vi "Periodic Tasks.vi"(8 "error in":errorcluster) -> ()   [LabVIEW 2014]
doc: "This VI runs in parallel to other tasks. It can contain as many user-defined periodic loops as you need. These can carry out PID or other sorts of timed response."
uses:
  <vilib>/Rock Robotics/SystemInterfaces/Utilities/FPGA_UtilitiesLED Source.ctl
  <vilib>/Rock Robotics/SystemInterfaces/Utilities/FPGA_UtilitiesLED State.ctl
  <vilib>/Rock Robotics/WPI/Compressor/WPI_CompressorGetSetRefNum.vi
  Robot Global Data.vi
  <vilib>/Rock Robotics/WPI/Relay/WPI_RelayValue.ctl
panel:
  out "Accel":dbl[](graph)=[0.0, 0.004] caption="Acceleration"
  in  "Blink Time (ms)":i32=2000
  in  "Thresh":dbl=1.0 caption="Acceleration Threshold"
  in  "Blink Speed":dbl=157.0 format="%#_13g"
  out "Color":u32(colorbox)=16728064
  in  "Speed":dbl=5.0 format="%#_13g"
  in  "Saturation":dbl(slide)=1.0 scale=0.0..1.0
  in  "Value":dbl(slide)=1.0 scale=0.0..1.0
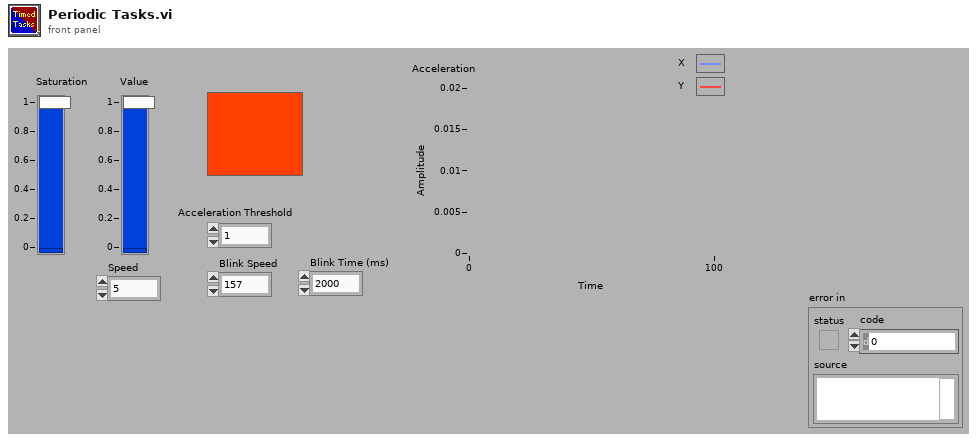
[diagram p1: front panel]
types:
  T1 = typedef "LEDStripRef.ctl" = cluster{"PWM Rate (Hz)":sgl, "Max Duty Cycle":sgl, "DigitalOutputRed":T2, "DigitalOutputGreen":T2, "DigitalOutputBlue":T2, "DevStatus":errorcluster}
  T2 = typedef "WPI_DigitalOutputDevRef.ctl" = cluster{"Digital Module":T3, "DIO Channel":T4, "DevStatus":errorcluster}
  T3 = typedef "FPGA_TypedefDigitalModule.ctl" = enum16{"Digital Module 1", "Digital Module 2"}
  T4 = typedef "FPGA_DIOChannel.ctl" = enum8{"DIO 1", "DIO 2", "DIO 3", "DIO 4", "DIO 5", "DIO 6", "DIO 7", "DIO 8", "DIO 9", "DIO 10", "DIO 11", "DIO 12", "DIO 13", "DIO 14", "Invalid"}
  T5 = typedef "WPI_I2CDevRef.ctl" = cluster{"DevStatus":errorcluster, "Digital Module":T3, "Device Address":u8}
  T6 = typedef "WPI_DigitalInputDevRef.ctl" = cluster{"DevStatus":errorcluster, "DIO Channel":T4, "Digital Module":T3}
  T7 = typedef "WPI_DriverStationRobotMode2.ctl" = enum16{"Autonomous Disabled", "Autonomous Enabled", "Teleop Disabled", "Teleop Enabled", "Disconnected", "Finish", "Test Disabled", "Test Enabled"}
  T8 = typedef "WPI_DriverStationAllianceInfo.ctl" = enum16{"Red", "Blue", "Invalid"}
  T9 = typedef "FPGA_UtilitiesLED State.ctl" = enum16{"Off", "On", "Toggle"}
  T10 = typedef "FPGA_UtilitiesLED Source.ctl" = enum16{"User LED", "FPGA LED"}
  T11 = typedef "WPI_CompressorDevRef.ctl" = cluster{"DevStatus":errorcluster, "DigitalInputDevRef":T6, "RelayDevRef":T12}
  T12 = typedef "WPI_RelayDevRef.ctl" = cluster{"DevStatus":errorcluster, "Relay Channel":T13, "Digital Module":T3, "Relay Direction":T14}
  T13 = typedef "FPGA_DIORelayChannel.ctl" = enum8{"Relay 1", "Relay 2", "Relay 3", "Relay 4", "Relay 5", "Relay 6", "Relay 7", "Relay 8", "Invalid"}
  T14 = typedef "WPI_RelayDirection.ctl" = enum16{"Both directions", "Forward only", "Reverse only"}
  T15 = typedef "WPI_RelayValue.ctl" = enum16{"Off", "On", "Forward", "Reverse"}
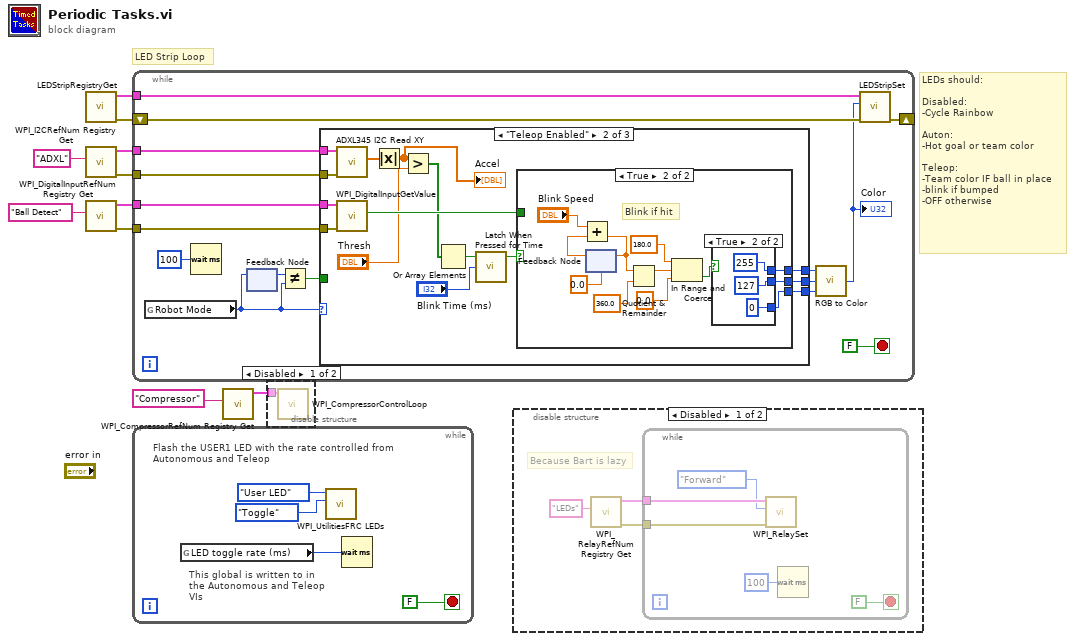
[diagram p0: block diagram]
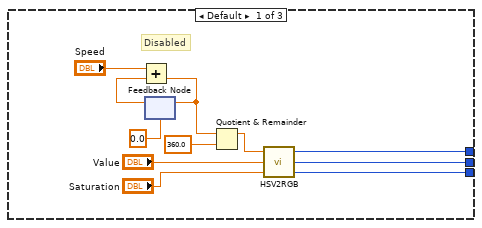
[diagram p4: hidden frame]
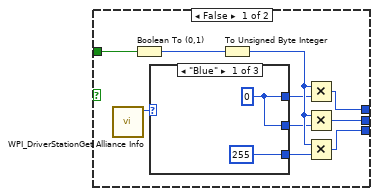
[diagram p5: hidden frame]
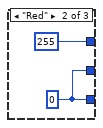
[diagram p6: hidden frame]
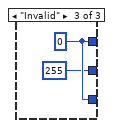
[diagram p7: hidden frame]
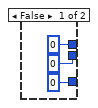
[diagram p8: hidden frame]
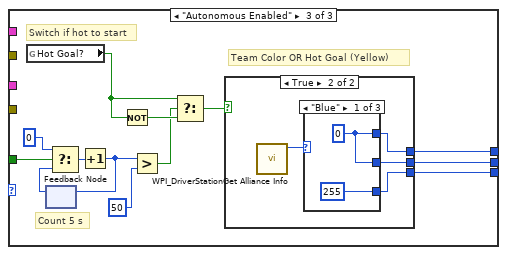
[diagram p9: hidden frame]
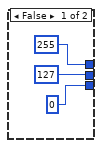
[diagram p10: hidden frame]
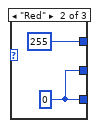
[diagram p11: hidden frame]
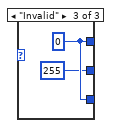
[diagram p12: hidden frame]
diagram:
  # "LEDs should:\n\nDisabled:\n-Cycle Rainbow\n\nAuton: \n-Hot goal or team color\n\nTeleop:\n-Team color IF ball in place\n-blink if bumped\n-OFF otherwise"
  # "LED Strip Loop"
  n1 = call "LEDStripRegistryGet.vi"() -> ("error out"=w7:errorcluster, "LEDStripRef out"=w8:T1)  [unwired: 10 in]
  n2 = call <vilib>:"WPI_I2CRefNum Registry Get.vi"("refnum name"="ADXL") -> ("error out"=w2:errorcluster, "I2CDevRef"=w3:T5)  [unwired: 9 in]
  n3 = call <vilib>:"WPI_DigitalInputRefNum Registry Get.vi"("refnum name"="Ball Detect") -> ("error out"=w4:errorcluster, "DigitalInputDevRef"=w5:T6)  [unwired: 9 in]
  n4 = while {
    tunnel: w8 -> [w24]
    shift-right: [w26] -> _
    shift-left: w7 -> [w23]
    tunnel: w5 -> [w18]
    tunnel: w4 -> [w17]
    tunnel: w3 -> [w12]
    tunnel: w2 -> [w11]
    stop <- FALSE stop-if-true
    n5 = global read "Robot Global Data.vi" "Robot Mode"() -> (w15:T7)
    n6 = Wait (ms)(milliseconds to wait=u32 100) -> ()  [unwired: 1 out]
    n7 = feedback-in #1(w15) -> ()
    n8 = feedback #1() -> (w16:T7)  [unwired: 1 in]
    n9 = Not Equal?(x=w16, y=w15) -> (x != y?=w14:bool)
    n10 = case shown="\"Teleop Enabled\"" w15 {
      tunnel: [w29 w49 w99] -> w22
      tunnel: [w28 w48 w98] -> w21
      tunnel: [w27 w47 w97] -> w20
      tunnel: w18 -> [_ w52 _]
      tunnel: w17 -> [_ w51 _]
      tunnel: w14 -> [_ _ w94]
      tunnel: w12 -> [_ w45 _]
      tunnel: w11 -> [_ w46 _]
      frame Default {
        # "Disabled"
        n11 = feedback #2(0.0) -> (w34:dbl)
        n12 = Add(x="Speed", y=w34) -> (x+y=w32:dbl)
        n13 = feedback-in #2(w32) -> ()
        n14 = Quotient & Remainder(x=w32, y=360.0) -> (x-y*floor(x/y)=w30:dbl)  [unwired: 1 out]
        n15 = call "HSV2RGB.vi"("Value"="Saturation", "Saturation"="Value", "Hue"=w30) -> ("Blue"=w27:u8, "Green"=w28:u8, "Red"=w29:u8)
      }
      frame "Teleop Enabled" {
        n16 = call "ADXL345 I2C Read XY.vi"("error in"=w46, "I2CDevRef"=w45) -> ("Acceleration XY"=w44:dbl[])  [unwired: 7 in, 2 out]
        n17 = call <vilib>:"WPI_DigitalInputGetValue.vi"("error in (no error)"=w51, "DigitalInputDevRef"=w52) -> ("Value"=w50:bool)  [unwired: 7 in, 2 out]
        n18 = Absolute Value(x=w44) -> (abs(x)=w38:dbl[])
        "Accel" <- w38
        n19 = Greater?(x=w38, y="Thresh") -> (0:w42:bool[])
        n20 = Or Array Elements(Boolean array=w42) -> (logical OR=w41:bool)
        n21 = call "Latch When Pressed for Time.vi"("Time (ms)"="Blink Time (ms)", "Input"=w41) -> ("Latched Output"=w40:bool)  [unwired: 3 in]
        n22 = case shown="True" w40 {
          tunnel: w50 -> [w62 _]
          tunnel: [w61 w70] -> w49
          tunnel: [w60 w71] -> w48
          tunnel: [w58 w69] -> w47
          frame False {
            n23 = call <vilib>:"WPI_DriverStationGet Alliance Info.vi"() -> ("Alliance"=w53:T8)  [unwired: 10 in, 1 out]
            n24 = Boolean To (0,1)(Boolean=w62) -> (0, 1=w59:i16)
            n25 = case shown="\"Blue\"" w53 {
              tunnel: [w63 u8 255 w68] -> w56
              tunnel: [u8 255 w65 w68] -> w55
              tunnel: [w63 w65 u8 255] -> w54
              frame "Blue" {
                w63 = u8 0
              }
              frame "Red" {
                w65 = u8 0
              }
              frame "Invalid" {
                w68 = u8 0
              }
            }
            n26 = To Unsigned Byte Integer(number=w59) -> (unsigned 8bit integer=w57:u8)
            n27 = Multiply(x=w57, y=w56) -> (x*y=w61:u8)
            n28 = Multiply(x=w57, y=w54) -> (x*y=w60:u8)
            n29 = Multiply(x=w57, y=w55) -> (x*y=w58:u8)
          }
          frame True {
            # "Blink if hit"
            n30 = feedback #3(0.0) -> (w79:dbl)
            n31 = Add(x="Blink Speed", y=w79) -> (x+y=w77:dbl)
            n32 = feedback-in #3(w77) -> ()
            n33 = Quotient & Remainder(x=w77, y=360.0) -> (x-y*floor(x/y)=w75:dbl)  [unwired: 1 out]
            n34 = In Range and Coerce(upper limit=180.0, x=w75, lower limit=0.0) -> (In Range?=w72:bool)  [unwired: 1 out]
            n35 = case shown="True" w72 {
              tunnel: [u8 0 u8 127] -> w71
              tunnel: [u8 0 u8 255] -> w70
              tunnel: [u8 0 u8 0] -> w69
              frame False {
              }
              frame True {
              }
            }
          }
        }
      }
      frame "Autonomous Enabled" {
        # "Switch if hot to start"
        # "Count 5 s"
        # "Team Color OR Hot Goal (Yellow)"
        n36 = global read "Robot Global Data.vi" "Hot Goal?"() -> (w88:bool)
        n37 = feedback #4() -> (w92:i32)  [unwired: 1 in]
        n38 = Select(t=0, s=w94, f=w92) -> (s? t:f=w91:i32)
        n39 = Increment(x=w91) -> (x+1=w90:i32)
        n40 = feedback-in #4(w90) -> ()
        n41 = Not(x=w88) -> (.not. x?=w96:bool)
        n42 = Greater?(x=w90, y=50) -> (0:w87:bool)
        n43 = Select(t=w88, s=w87, f=w96) -> (s? t:f=w95:bool)
        n44 = case shown="True" w95 {
          tunnel: [u8 255 w106] -> w99
          tunnel: [u8 127 w105] -> w98
          tunnel: [u8 0 w104] -> w97
          frame False {
          }
          frame True {
            n45 = call <vilib>:"WPI_DriverStationGet Alliance Info.vi"() -> ("Alliance"=w103:T8)  [unwired: 10 in, 1 out]
            n46 = case shown="\"Blue\"" w103 {
              tunnel: [w107 u8 255 w112] -> w106
              tunnel: [u8 255 w109 w112] -> w104
              tunnel: [w107 w109 u8 255] -> w105
              frame "Blue" {
                w107 = u8 0
              }
              frame "Red" {
                w109 = u8 0
              }
              frame "Invalid" {
                w112 = u8 0
              }
            }
          }
        }
      }
    }
    n47 = call <vilib>:"RGB to Color.vi"("B"=w20, "G"=w21, "R"=w22) -> ("Color"=w13:u32)
    "Color" <- w13
    n48 = call "LEDStripSet.vi"("error in"=w23, "Color"=w13, "LEDStripRef in"=w24) -> ("error out"=w26:errorcluster)  [unwired: 7 in, 1 out]
  }
  n49 = while {
    stop <- FALSE stop-if-true
    # "This global is written to in the Autonomous and Teleop VIs"
    # "Flash the USER1 LED with the rate controlled from Autonomous and Teleop"
    n50 = global read "Robot Global Data.vi" "LED toggle rate (ms)"() -> (w113:u32)
    n51 = call <vilib>:"WPI_UtilitiesFRC LEDs.vi"("State"=FPGA_UtilitiesLED_State."Toggle", "LED Type"=FPGA_UtilitiesLED_Source."User LED") -> ()  [unwired: 1 in, 9 out]
    n52 = Wait (ms)(milliseconds to wait=w113) -> ()  [unwired: 1 out]
  }
  n53 = call <vilib>:"WPI_CompressorRefNum Registry Get.vi"("refnum name"="Compressor") -> ("CompressorDevRef"=w9:T11)  [unwired: 9 in, 1 out]
  n54 = disable-structure shown="Disabled" {
    disable-tunnel: w9 -> [w117 _]
    frame Disabled {
      n55 = call <vilib>:"WPI_CompressorControlLoop.vi"("CompressorDevRef"=w117) -> ()  [unwired: 11 in]
    }
    frame Enabled {
    }
  }
  n56 = disable-structure shown="Disabled" {
    frame Disabled {
      # "Because Bart is lazy"
      n57 = call <vilib>:"WPI_RelayRefNum Registry Get.vi"("refnum name"="LEDs") -> ("error out"=w118:errorcluster, "RelayDevRef"=w119:T12)  [unwired: 9 in]
      n58 = while {
        tunnel: w119 -> [w125]
        tunnel: w118 -> [w123]
        stop <- FALSE stop-if-true
        n59 = call <vilib>:"WPI_RelaySet.vi"("error in (no error)"=w123, "RelayValue"=WPI_RelayValue."Forward", "RelayDevRef"=w125) -> ()  [unwired: 7 in, 2 out]
        n60 = Wait (ms)(milliseconds to wait=u32 100) -> ()  [unwired: 1 out]
      }
    }
    frame Enabled {
    }
  }
